vi "Save ROI.vi"() -> ()   [LabVIEW 2022 SP3]
panel:
  out "Global Rectangle":i32[](array[numeric])=[300, 243, 582, 509]
  out "No. of Images":i32
  out "Image":i32
  in  "OK Button":bool
  out "ROI Image":T1(plugin-control)
  out "Source Image":T1(plugin-control)
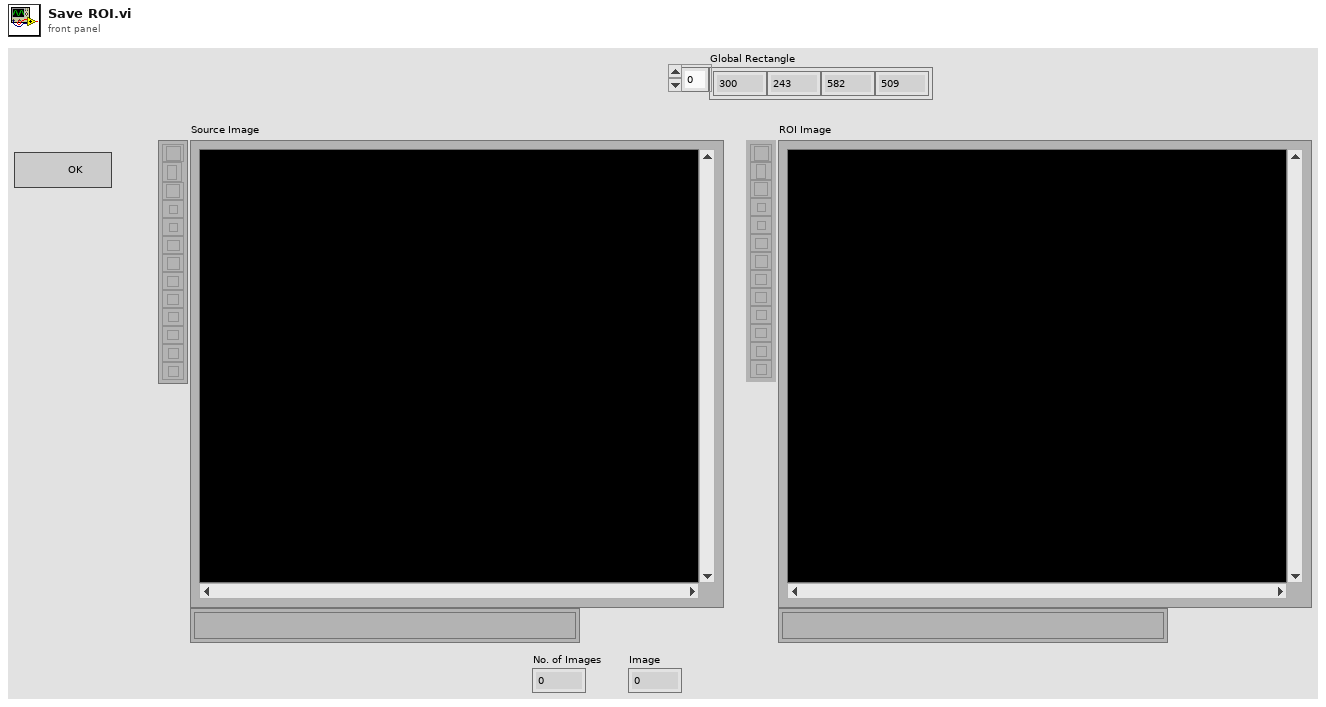
[diagram p1: front panel]
types:
  T1 = typedef "IMAQ Image.ctl" = refnum<image>
  T2 = typedef "Image Type" = u32
  T3 = cluster{"Global Rectangle":i32[], "Contours":cluster{"Contour Type":u32, "ROI Type":u32, "Points":i32[]}[]}
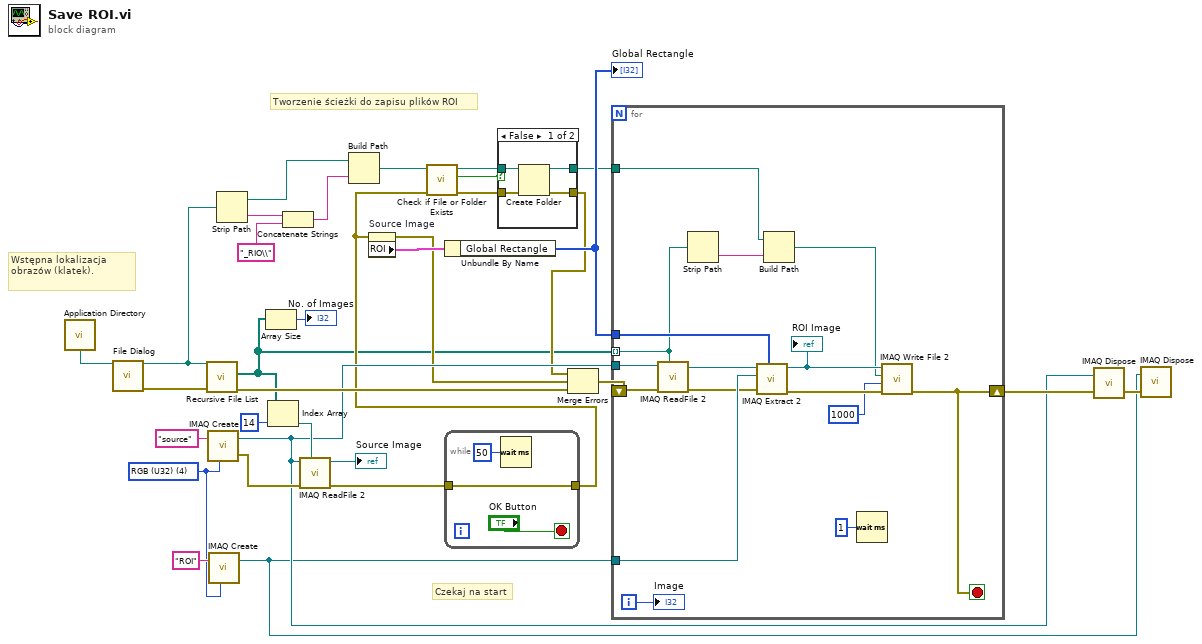
[diagram p0: block diagram]
diagram:
  w20 = T2 4 items=["Grayscale (U8)", "Grayscale (I16)", "Grayscale (SGL)", "Complex (CSG)", "RGB (U32)", "HSL (U32)", "RGB (U64)", "Grayscale (U16)"] ("Image Type")
  # "Tworzenie ścieżki do zapisu plików ROI"
  # "Czekaj na start"
  # "Wstępna lokalizacja obrazów (klatek)."
  n1 = call <vilib>:"Application Directory.vi"() -> ("Application Directory"=w33:path)
  n2 = call "File Dialog"("start path"=w33) -> ("selected path"=w4:path, "error out"=w32:errorcluster)  [unwired: 11 in, 2 out]
  n3 = call <vilib>:"Recursive File List.vi"("error in (no error)"=w32, "Folder Path"=w4) -> ("error out"=w30:errorcluster, "All Files in Dir"=w2:path[])  [unwired: 5 in, 3 out]
  n4 = call "IMAQ Create"("Image Name"="source", "Image Type"=w20) -> ("New Image"=w17:T1, "error out"=w29:errorcluster)  [unwired: 3 in]
  n5 = call "IMAQ Create"("Image Name"="ROI", "Image Type"=w20) -> ("New Image"=w16:T1)  [unwired: 3 in, 1 out]
  n6 = Strip Path(path=w4) -> (stripped path=w3:path, name=w14:string)
  n7 = Array Size(array=w2) -> (size(s)=→"No. of Images":i32)
  n8 = Index Array(array=w2, index=14) -> (element=w27:path)
  n9 = Concatenate Strings(w14, "_RIO\\") -> (w12:string)
  n10 = call "IMAQ ReadFile 2"("File Path"=w27, "error in (no error)"=w29, "Image"=w17) -> ("error out"=w23:errorcluster, "Image Out"=→"Source Image":T1)  [unwired: 4 in, 3 out]
  n11 = Build Path(base path=w3, name or relative path=w12) -> (appended path=w8:path)
  n12 = while {
    tunnel: w23 -> [w34]
    tunnel: [w34] -> w7
    stop <- "OK Button" stop-if-true
    n13 = Wait (ms)(milliseconds to wait=u32 50) -> ()  [unwired: 1 out]
  }
  n14 = property on="Source Image" class="ImageControl"(error in=w7) -> (error out=w15:errorcluster, "ROI"=w25:T3)  [unwired: 1 in, 1 out]
  n15 = call <vilib>:"Check if File or Folder Exists.vi"("error in (no error)"=w7, "path"=w8) -> ("error out"=w10:errorcluster, "file or folder exists?"=w9:bool, "dup path"=w11:path)  [unwired: 7 in]
  n16 = Unbundle By Name(w25) -> ("Global Rectangle"=w22:i32[])
  "Global Rectangle" <- w22
  n17 = case shown="False" w9 {
    tunnel: w10 -> [w40 w41]
    tunnel: w11 -> [w39 w42]
    tunnel: [w38 w42] -> w5
    tunnel: [w37 w41] -> w6
    frame False {
      n18 = Create Folder(path (use dialog)=w39, error in=w40) -> (created path=w38:path, error out=w37:errorcluster)  [unwired: 1 in, 1 out]
    }
    frame True {
    }
  }
  n19 = Merge Errors(w6, w15, w30) -> (w24:errorcluster)
  n20 = for {
    tunnel: w2 -> [w48] mode=indexing
    tunnel: w17 -> [w58]
    tunnel: w22 -> [w56]
    tunnel: w16 -> [w54]
    shift-right: [w51] -> w19
    shift-left: w24 -> [w57]
    tunnel: w5 -> [w47]
    i -> [w44]
    stop <- w51 stop-if-true
    n21 = call "IMAQ ReadFile 2"("File Path"=w48, "error in (no error)"=w57, "Image"=w58) -> ("error out"=w53:errorcluster, "Image Out"=w55:T1)  [unwired: 4 in, 3 out]
    n22 = Strip Path(path=w48) -> (name=w46:string)  [unwired: 1 out]
    n23 = call "IMAQ Extract 2"("Optional Rectangle"=w56, "error in (no error)"=w53, "Image Dst"=w54, "Image Src"=w55) -> ("error out"=w52:errorcluster, "Image Dst Out"=w49:T1)  [unwired: 6 in]
    "ROI Image" <- w49
    n24 = Build Path(base path=w47, name or relative path=w46) -> (appended path=w45:path)
    n25 = Wait (ms)(milliseconds to wait=u32 1) -> ()  [unwired: 1 out]
    n26 = call-poly "IMAQ Write File 2"("error in (no error)"=w52, "Image Quality"=u32 1000, "File Path"=w45, "Image"=w49) -> ("error out"=w51:errorcluster)  [unwired: 6 in, 1 out]
    "Image" <- w44
  }
  n27 = call "IMAQ Dispose"("Image"=w17, "error in (no error)"=w19) -> ("error out"=w18:errorcluster)  [unwired: 4 in]
  n28 = call "IMAQ Dispose"("Image"=w16, "error in (no error)"=w18) -> ()  [unwired: 4 in, 1 out]
